vi "DriveNetwork.vi"(8 "error in (no error)":errorcluster) -> (0 "error out":errorcluster)   [LabVIEW 2020]
doc: "Network for Drive\n\nInputs:\n -- Error in -- Error cluster -- propagated error input\n\nOutputs:\n -- Error out -- Error cluster -- progated error output"
uses:
  <vilib>/Rock Robotics/WPI/ThirdParty/JAS_Junk/TrajLib/LinearFilter_ResetToValue.vi
  <vilib>/Rock Robotics/WPI/ThirdParty/JAS_Junk/TrajLib/LinearFilter_Calculate.vi
  DriveGlobal.vi
  <vilib>/Rock Robotics/WPI/ThirdParty/JAS_Junk/TrajLib/LinearFilter_MovingAverage.vi
  <vilib>/Rock Robotics/WPI/ThirdParty/JAS_Junk/TrajLib/LinearFilter_LowPassBW1.vi
  <vilib>/Rock Robotics/WPI/ThirdParty/JAS_Junk/TrajLib/LinearFilter_LowPassBW2.vi
  <vilib>/Rock Robotics/WPI/ThirdParty/JAS_Junk/TrajLib/LinearFilter_HighPassBW1.vi
  <vilib>/Rock Robotics/WPI/ThirdParty/JAS_Junk/TrajLib/LinearFilter_HighPassBW2.vi
  <vilib>/Rock Robotics/Network Tables/NT Write Number.vi
  <vilib>/Rock Robotics/WPI/ThirdParty/JAS_Junk/TrajLib/Trajectory_Library.lvlib
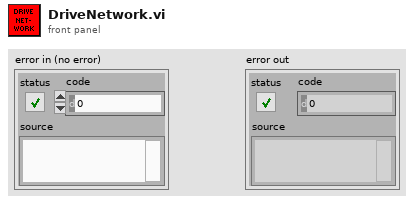
[diagram p1: front panel]
types:
  T1 = enum16{"Moving Average", "Low Pass 1st Order Butterworth", "Low Pass 2nd Order Butterworth", "High Pass 1st Order Butterworth", "High Pass 2nd Order Butterworth"}
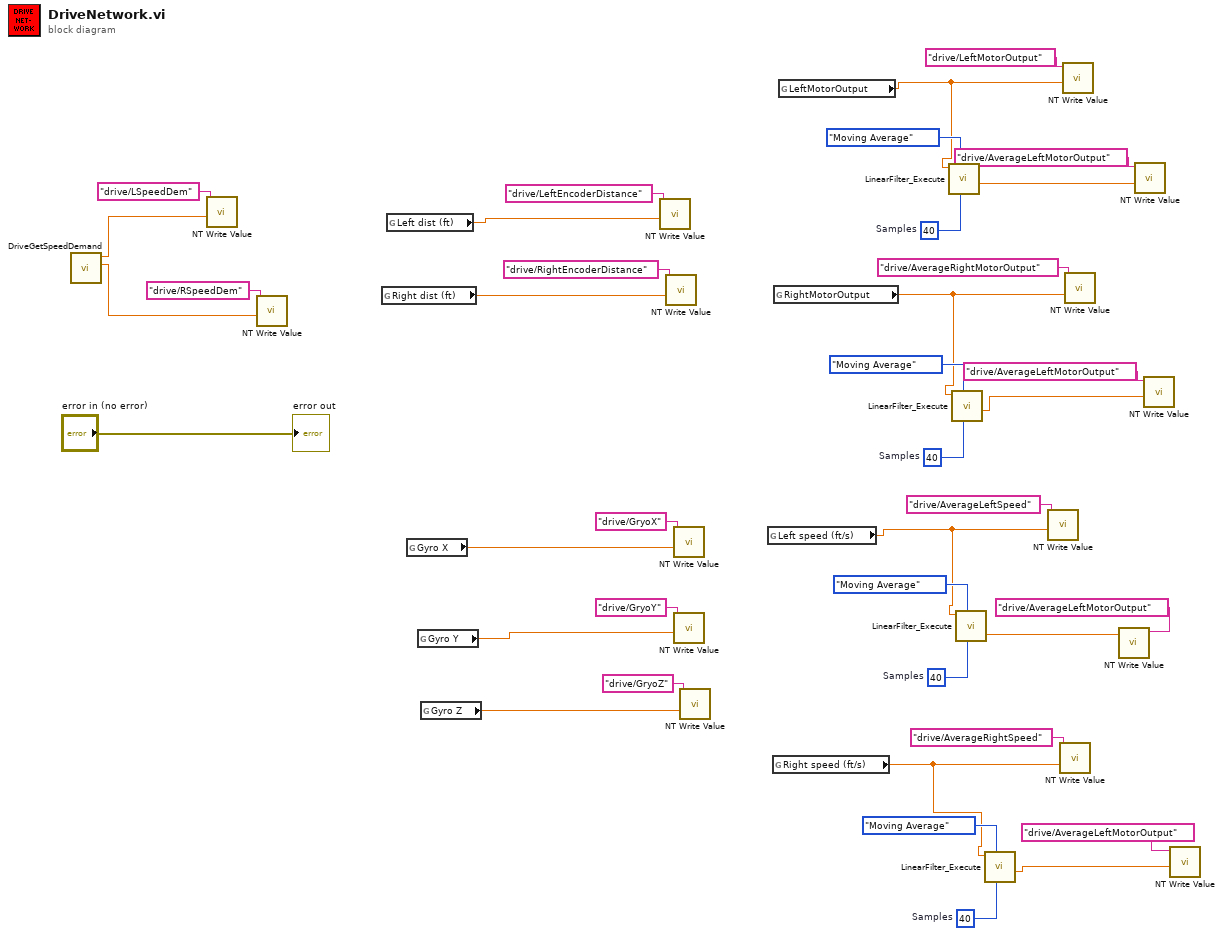
[diagram p0: block diagram]
diagram:
  w14 = 40  # Samples
  w16 = 40  # Samples
  w18 = 40  # Samples
  w20 = 40  # Samples
  n1 = call "DriveGetSpeedDemand.vi"() -> ("RSpeedDemand (ft/s)"=w35:dbl, "LSpeedDemand (ft/s)"=w37:dbl)  [unwired: 10 in]
  n2 = call-poly <vilib>:"NT Write Value.vi"("value"=w37, "name"="drive/LSpeedDem") -> ()  [unwired: 9 in, 1 out]
  n3 = call-poly <vilib>:"NT Write Value.vi"("value"=w35, "name"="drive/RSpeedDem") -> ()  [unwired: 9 in, 1 out]
  n4 = global read "DriveGlobal.vi" "Right dist (ft)"() -> (w30:dbl)
  n5 = global read "DriveGlobal.vi" "Left dist (ft)"() -> (w29:dbl)
  n6 = global read "DriveGlobal.vi" "Gyro X"() -> (w23:dbl)
  n7 = global read "DriveGlobal.vi" "Gyro Y"() -> (w24:dbl)
  n8 = global read "DriveGlobal.vi" "Gyro Z"() -> (w25:dbl)
  n9 = call-poly <vilib>:"NT Write Value.vi"("value"=w29, "name"="drive/LeftEncoderDistance") -> ()  [unwired: 9 in, 1 out]
  n10 = call-poly <vilib>:"NT Write Value.vi"("value"=w30, "name"="drive/RightEncoderDistance") -> ()  [unwired: 9 in, 1 out]
  n11 = call-poly <vilib>:"NT Write Value.vi"("value"=w23, "name"="drive/GryoX") -> ()  [unwired: 9 in, 1 out]
  n12 = call-poly <vilib>:"NT Write Value.vi"("value"=w24, "name"="drive/GryoY") -> ()  [unwired: 9 in, 1 out]
  n13 = call-poly <vilib>:"NT Write Value.vi"("value"=w25, "name"="drive/GryoZ") -> ()  [unwired: 9 in, 1 out]
  n14 = global read "DriveGlobal.vi" "Left speed (ft/s)"() -> (w7:dbl)
  n15 = global read "DriveGlobal.vi" "Right speed (ft/s)"() -> (w8:dbl)
  n16 = global read "DriveGlobal.vi" "RightMotorOutput"() -> (w6:dbl)
  n17 = global read "DriveGlobal.vi" "LeftMotorOutput"() -> (w5:dbl)
  n18 = call <vilib>:"LinearFilter_Execute.vi"("Samples"=w14, "Filter Type"=T1."Moving Average", "Input"=w5) -> ("Output"=w4:dbl)  [unwired: 7 in, 1 out]
  n19 = call <vilib>:"LinearFilter_Execute.vi"("Samples"=w16, "Filter Type"=T1."Moving Average", "Input"=w6) -> ("Output"=w3:dbl)  [unwired: 7 in, 1 out]
  n20 = call <vilib>:"LinearFilter_Execute.vi"("Samples"=w18, "Filter Type"=T1."Moving Average", "Input"=w7) -> ("Output"=w2:dbl)  [unwired: 7 in, 1 out]
  n21 = call <vilib>:"LinearFilter_Execute.vi"("Samples"=w20, "Filter Type"=T1."Moving Average", "Input"=w8) -> ("Output"=w1:dbl)  [unwired: 7 in, 1 out]
  n22 = call-poly <vilib>:"NT Write Value.vi"("value"=w7, "name"="drive/AverageLeftSpeed") -> ()  [unwired: 9 in, 1 out]
  n23 = call-poly <vilib>:"NT Write Value.vi"("value"=w8, "name"="drive/AverageRightSpeed") -> ()  [unwired: 9 in, 1 out]
  n24 = call-poly <vilib>:"NT Write Value.vi"("value"=w5, "name"="drive/LeftMotorOutput") -> ()  [unwired: 9 in, 1 out]
  n25 = call-poly <vilib>:"NT Write Value.vi"("value"=w6, "name"="drive/AverageRightMotorOutput") -> ()  [unwired: 9 in, 1 out]
  n26 = call-poly <vilib>:"NT Write Value.vi"("value"=w2, "name"="drive/AverageLeftMotorOutput") -> ()  [unwired: 9 in, 1 out]
  n27 = call-poly <vilib>:"NT Write Value.vi"("value"=w4, "name"="drive/AverageLeftMotorOutput") -> ()  [unwired: 9 in, 1 out]
  n28 = call-poly <vilib>:"NT Write Value.vi"("value"=w3, "name"="drive/AverageLeftMotorOutput") -> ()  [unwired: 9 in, 1 out]
  n29 = call-poly <vilib>:"NT Write Value.vi"("value"=w1, "name"="drive/AverageLeftMotorOutput") -> ()  [unwired: 9 in, 1 out]
  "error out" <- "error in (no error)"
